vi "Get Sink Terminals from Source.vi"(8 "error in (no error)":errorcluster, 11 "Source Terminal":refnum<vi>) -> (0 "error out":errorcluster, 3 "Sink Terminals":refnum<vi>[](array[refnum]))   [LabVIEW 2013, in "JKI State Machine API.lvlib" / "JKI SM.lvclass"]
uses:
  JKI SM/JKI SM.lvclass
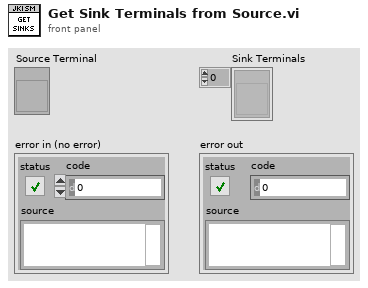
[diagram p1: front panel]
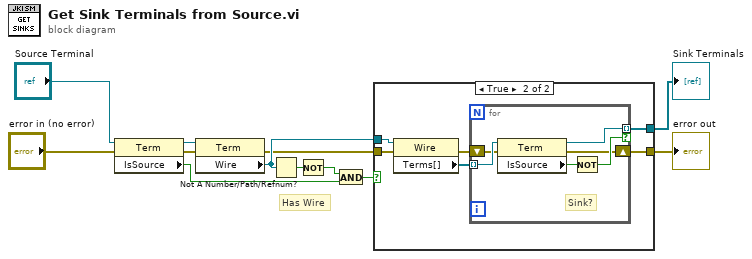
[diagram p0: block diagram]
diagram:
  # "Has Wire"
  n1 = property class="Term"(reference="Source Terminal", error in="error in (no error)") -> (reference out=w4:refnum<vi>, error out=w5:errorcluster, "IsSource"=w8:bool)
  n2 = property class="Term"(reference=w4, error in=w5) -> (error out=w1:errorcluster, "Wire"=w9:refnum<vi>)  [unwired: 1 out]
  n3 = Not A Number/Path/Refnum?(number/path/refnum=w9) -> (NaN/Path/Refnum?=w6:bool)
  n4 = Not(x=w6) -> (.not. x?=w7:bool)
  n5 = And(x=w7, y=w8) -> (x .and. y?=w2:bool)
  n6 = case shown="True" w2 {
    tunnel: [w13 w18] -> w12
    tunnel: [_ w17] -> w10
    tunnel: w9 -> [_ w15]
    tunnel: w1 -> [w13 w14]
    frame False {
    }
    frame True {
      n7 = property class="Wire"(reference=w15, error in=w14) -> (error out=w19:errorcluster, "Terms[]"=w16:refnum<vi>[])  [unwired: 1 out]
      n8 = for {
        tunnel: w16 -> [w25] mode=indexing
        tunnel: [w23] -> w17 mode=indexing if=w22
        shift-right: [w21] -> w18
        shift-left: w19 -> [w20]
        # "Sink?"
        n9 = property class="Term"(reference=w25, error in=w20) -> (reference out=w23:refnum<vi>, error out=w21:errorcluster, "IsSource"=w24:bool)
        n10 = Not(x=w24) -> (.not. x?=w22:bool)
      }
    }
  }
  "error out" <- w12
  "Sink Terminals" <- w10
